vi "Configure Spurious Emission (Segment Function Setup).vi"(0 "VISA resource name":refnum<visa-resource-name>, 1 "Spurious Table Number (1)":i32=1 min=1 max=20, 2 "Spurious Load Correction Table Recall (F:Disable)":bool, 5 "Spurious Correction Table":T1={"Segment Number (1)"=1, "Filename (FileName)"="FileName", "Device (D)"="D"} {"Segment Number (1)" min=1 max=20}, 7 "Spurious Pause Mode":i32[](array[ring]) items=["Off", "On"], 9 "Spurious Segment Mode":i32[](array[ring]) items=["Off", "On"], 11 "error in (no error)":errorcluster) -> (4 "VISA resource name out":refnum<visa-resource-name>, 15 "error out":errorcluster)   [LabVIEW 2020, in "Anritsu Signal Analyzer Series.lvlib"]
doc: "Configures the function for segment parameter of Spurious Emission measurement."
uses:
  Anritsu Signal Analyzer Series.lvlib
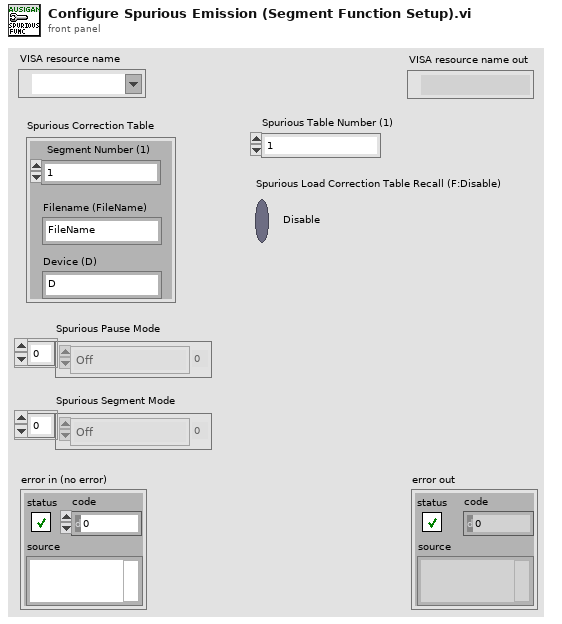
[diagram p1: front panel]
types:
  T1 = cluster{"Segment Number (1)":i32, "Filename (FileName)":string, "Device (D)":string}
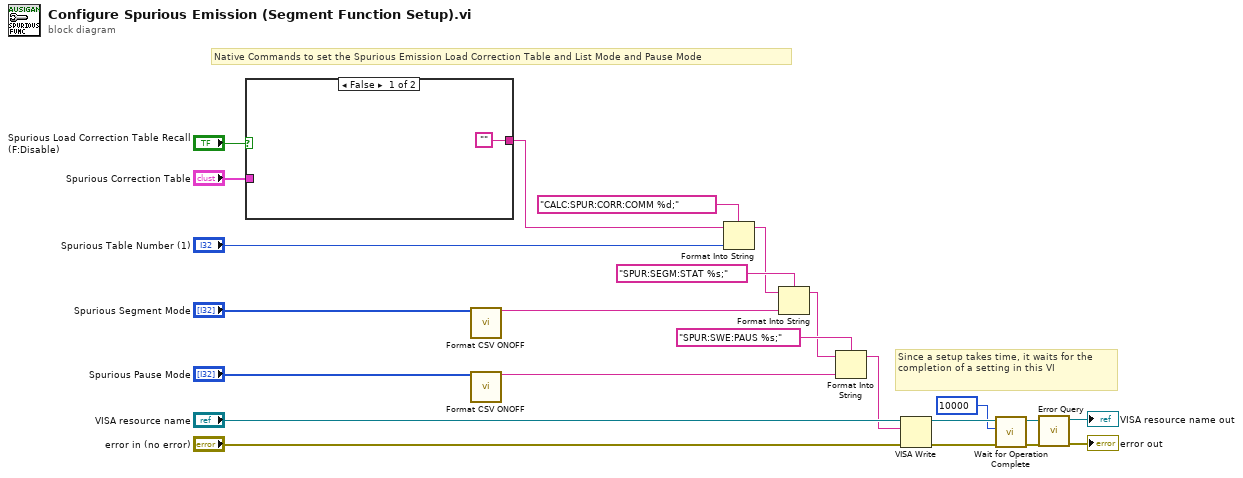
[diagram p0: block diagram]
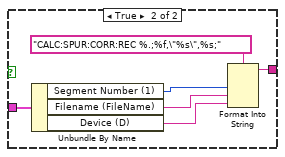
[diagram p2: hidden frame]
diagram:
  # "Since a setup takes time, it waits for the completion of a setting in this VI"
  # "Native Commands to set the Spurious Emission Load Correction Table and List Mode and Pause Mode"
  n1 = case shown="False" "Spurious Load Correction Table Recall (F:Disable)" {
    tunnel: "Spurious Correction Table" -> [_ w30]
    tunnel: ["" w25] -> w13
    frame False {
    }
    frame True {
      n2 = Unbundle By Name(w30) -> ("Segment Number (1)"=w28:i32, "Filename (FileName)"=w27:string, "Device (D)"=w26:string)
      n3 = Format Into String(format string="CALC:SPUR:CORR:REC %.;%f,\"%s\",%s;" ("_Command"), w28, w27, w26) -> (resulting string=w25:string)  [unwired: 2 in, 1 out]
    }
  }
  n4 = call "Format CSV ONOFF.vi"("Data_In"="Spurious Segment Mode") -> ("Data_out"=w7:string)  [unwired: 14 in]
  n5 = call "Format CSV ONOFF.vi"("Data_In"="Spurious Pause Mode") -> ("Data_out"=w5:string)  [unwired: 14 in]
  n6 = Format Into String(format string="CALC:SPUR:CORR:COMM %d;", initial string=w13, "Spurious Table Number (1)") -> (resulting string=w12:string)  [unwired: 1 in, 1 out]
  n7 = Format Into String(format string="SPUR:SEGM:STAT %s;" ("_CommandSet"), initial string=w12, w7) -> (resulting string=w11:string)  [unwired: 1 in, 1 out]
  n8 = Format Into String(format string="SPUR:SWE:PAUS %s;" ("_CommandSet"), initial string=w11, w5) -> (resulting string=w10:string)  [unwired: 1 in, 1 out]
  n9 = VISA Write(VISA resource name="VISA resource name", write buffer=w10, error in (no error)="error in (no error)") -> (VISA resource name out=w4:refnum<visa-resource-name>, error out=w3:errorcluster)  [unwired: 1 out]
  n10 = call "Wait for Operation Complete.vi"("error in (no error)"=w3, "Maximum Time (10000mSec)"=10000, "VISA resource name"=w4) -> ("error out"=w8:errorcluster, "VISA resource name out"=w9:refnum<visa-resource-name>)  [unwired: 7 in]
  n11 = call "Error Query.vi"("error in (no error)"=w8, "VISA resource name"=w9) -> ("error out"=→"error out":errorcluster, "VISA resource name out"=→"VISA resource name out":refnum<visa-resource-name>)  [unwired: 6 in, 2 out]
